vi "FFT.vi"() -> ()   [LabVIEW 2020]
uses:
  <vilib>/Platform/TimedLoop/XDataNode/timing_clust.ctl
  <vilib>/Platform/TimedLoop/XDataNode/nitl_modes.ctl
  <vilib>/Platform/TimedLoop/XDataNode/wakeup.ctl
  <vilib>/rvi/Analysis/measure/FFT/simModelSupport/niFPGA FFT Streaming Sim Properties.ctl
  <vilib>/rvi/Analysis/measure/FFT/simModelSupport/niFPGA FFT Sim Stream Group Properties.ctl
  <vilib>/rvi/Analysis/measure/FFT/simModelSupport/niFPGA FFT Sim Types.ctl
  <vilib>/rvi/Analysis/measure/FFT/simModelSupport/niFpgaFFTSimArithmeticProperties.ctl
  <vilib>/rvi/Analysis/measure/FFT/simModelSupport/niFpgaFFTSimDfxp.ctl
  <vilib>/fxp/LVFixedPointQuantizationPolicyTypeDef.ctl
  <vilib>/rvi/Analysis/measure/FFT/XNode/niFpgaFFTButterflyDelays.ctl
  <vilib>/rvi/DataTransferAndStorage/Container/Common/niFpgaContainerGetUniqueNameForEmu.vi
  <vilib>/rvi/DataTransferAndStorage/Container/Common/niFpgaContainerSetEmuInfo.vi
  <vilib>/rvi/eio/common/nirviEmuReportErrorAndStop.vi
  <vilib>/rvi/interface/RandomDataEmulation/niFpgaRandomDataHandleErrors.vi
  <vilib>/rvi/DataTransferAndStorage/Container/Common/niFpgaContainerExecOnDevCompGetState.vi
  <vilib>/rvi/Emulation/niFpgaEmulationIsFPGAContextNoSignature.vi
  <vilib>/rvi/Emulation/niFpgaSctlEmulationGetInTimedLoop.vi
  <vilib>/rvi/errors/niFpgaSetErrorForExecOnDevCompSimple.vi
  <vilib>/rvi/FIFO/Fifo_Resource/nirvififoEmulationSetSize.vi
  <vilib>/rvi/FIFO/Fifo_Resource/nirviFifoEmulationQueueMgr.vi
  <instcachedir>/0/nirviFifoEmulationQueueMgr_E5CAEC123FF24DC58D834DCA3CDAA9B5.lvgen/nirviFifoEmulationQueueMgr_E5CAEC123FF24DC58D834DCA3CDAA9B5_008.vi
  <vilib>/rvi/FIFO/Fifo_Resource/nirvififoEmulationDetermineInputValidOut.vi
  <vilib>/rvi/FIFO/Fifo_Resource/nirvififoEmulationCreateLock.vi
  <vilib>/rvi/Emulation/niFpgaProcessEmulError.vi
  <vilib>/rvi/FIFO/Fifo_Resource/nirvififoEmulationObtainLock.vi
  <vilib>/rvi/FIFO/Fifo_Resource/nirvififoEmulationReleaseLock.vi
  <vilib>/rvi/occurrence/nirviWaitOnOccurrenceBase.vi
  <vilib>/rvi/errors/nirviReportUnexpectedCaseInternalError.vi
  <vilib>/rvi/errors/nirviReportUnexpectedCaseInternalError (U32).vi
  <vilib>/Utility/error.llb/Clear Errors.vi
  <vilib>/rvi/Emulation/niFpgaEmulationReportErrorSimple.vi
  <vilib>/rvi/Emulation/niFpgaGetClockAttributes.vi
  <vilib>/rvi/Emulation/niFpgaCriticalErrorInLSC.vi
  <vilib>/rvi/Analysis/measure/FFT/simModelSupport/niFpgaFFTSimModelStreamingCore.vi
  <vilib>/rvi/LocalResourceManager/LocalResourceManager.xnode
  <vilib>/rvi/DataTransferAndStorage/Container/XNode/niFpgaContainer.xnode
  <vilib>/rvi/interface/RandomDataEmulation/nirviRandomDataFpgaReadWriteTemplate.vi
  <vilib>/rvi/FIFO/Fifo_Resource/niFpgaFifoEmulationRefIn.vi
  <vilib>/Platform/TimedLoop/XDataNode/XDataNode.xnode
  <vilib>/rvi/Analysis/measure/FFT/XNode/niFpgaFFT.xnode
  <vilib>/rvi/FXPMathLib/FxpInterpret/XNode/nifxpmath_Interpret.xnode
  <vilib>/Platform/TimedLoop/XDataNode/XDNodeRunTimeDep.lvlib
panel:
  out "overflow":bool
  out "loop numbers for FFT":i32
  out "loop number for data collection":i32
  out "appended array":fxp<+/-,24,7>[](array[numeric])
  out "FFT time (uSec)":u32
  out "data collection time (uSec)":u32
  in  "auto stop":bool
  in  "FFT loop iterations":i32
  out "Element":fxp<+/-,24,7>
  in  "Loop number":i32
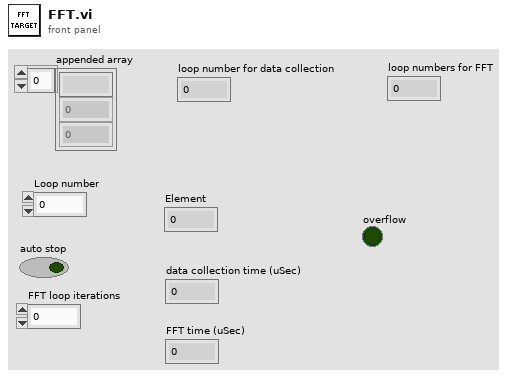
[diagram p1: front panel]
types:
  T1 = typedef "XDNodeRunTimeDep.lvlib/timing_clust.ctl" = cluster{"Expected End [f-1]":u64, "Actual End [f-1]":u64, "Finished Late? [f-1]":bool, "Expected End [i-1]":u64, "Actual End [i-1]":u64, "Finished Late? [i-1]":bool, "Expected Start [i]":u64, "Actual Start [i]":u64, "Expected Start [f]":u64, "Actual Start [f]":u64, "Source Name":string, "Structure Name":string, "Period":i64, "Deadline":i64, "Offset":i64, "Start":i64, "Priority":i32, "Timeout":i32, "Mode":T2, "Wakeup Reason":T3, "Error":errorcluster, "Source Type":string, "Secondary Source Type":string, "Global End Time":u64, "Global Start Time":u64, "Frame Duration":u64, "Iteration Duration":u64, "Assigned CPU":i32, "I/O Scan Engine Mode":u32}
  T2 = typedef "XDNodeRunTimeDep.lvlib/nitl_modes.ctl" = enum32{"No Change", "Process missed periods, maintain original phase", "Discard missed periods, maintain original phase", "Process missed periods, ignore original phase", "Discard missed periods, ignore original phase"}
  T3 = typedef "XDNodeRunTimeDep.lvlib/wakeup.ctl" = enum32{"Normal", "Aborted", "Asynchronous wakeup", "Timing source error", "Timed loop error", "Timeout"}
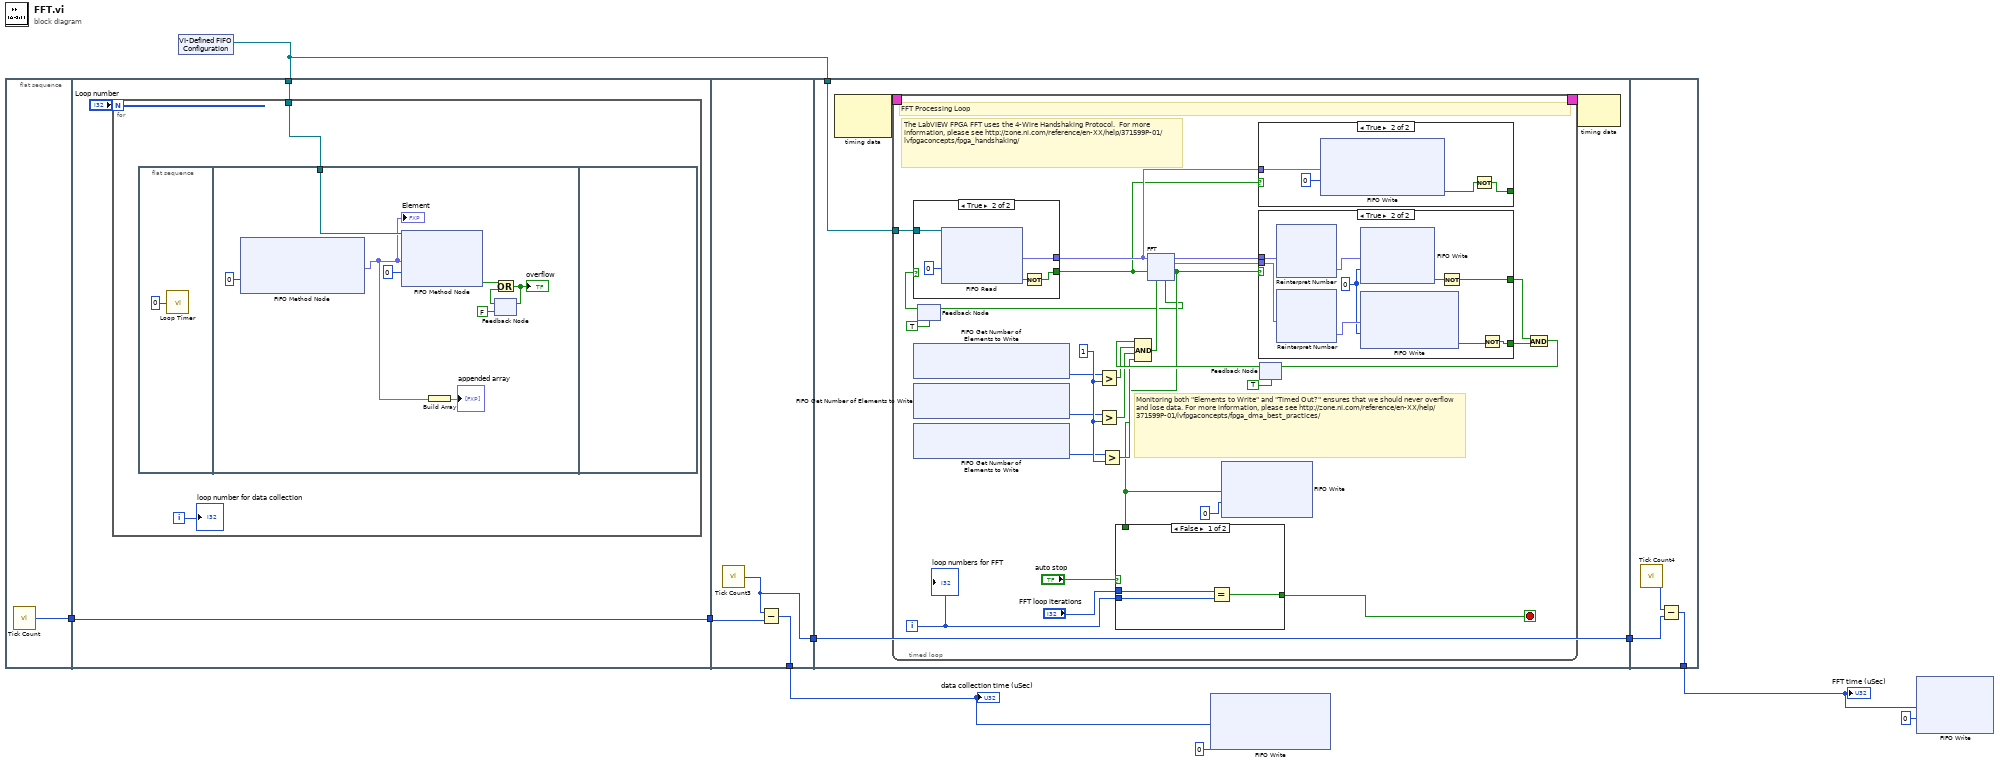
[diagram p0: block diagram]
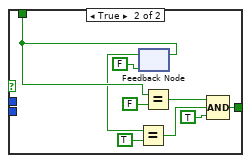
[diagram p2: hidden frame]
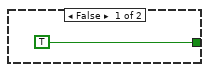
[diagram p3: hidden frame]
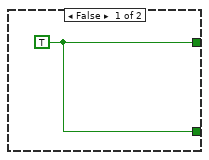
[diagram p4: hidden frame]
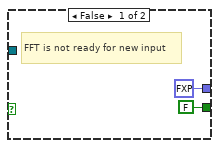
[diagram p5: hidden frame]
diagram:
  n1 = flat-sequence {
    tunnel: [w10] -> w9
    tunnel: w5 -> [w13]
    tunnel: w9 -> [w11]
    tunnel: [w11] -> w8
    tunnel: w8 -> [w28]
    tunnel: [w27] -> w4
    tunnel: [w26] -> w7
    tunnel: w5 -> [w30]
    tunnel: w7 -> [w29]
    tunnel: [w29] -> w6
    tunnel: w6 -> [w125]
    tunnel: [w124] -> w1
    frame #0 {
      n2 = call "Tick Count"() -> ("Tick Count(uSec)"=w10:u32)
    }
    frame #1 {
      n3 = for {
        N: "Loop number" -> [_]
        tunnel: w13 -> [w15]
        i -> [w14]
        n4 = flat-sequence {
          tunnel: w15 -> [w24]
          frame #0 {
            n5 = call "Loop Timer"("Count(mSec)"=u32 0) -> ()  [unwired: 1 out]
          }
          frame #1 {
            n6 = xnode ("FIFO Method Node")("Timeout"=0) -> ("Element"=w22:fxp<+/-,24,7>)  [unwired: 1 in, 2 out]
            "Element" <- w22
            n7 = xnode ("FIFO Method Node")("Element"=w22, "Timeout"=0, "FIFO In"=w24) -> ("Timed Out?"=w19:bool)  [unwired: 1 in, 2 out]
            n8 = Build Array(w22) -> (→"appended array":fxp<+/-,24,7>[])
            n9 = feedback #1(FALSE) -> (w18:bool)
            n10 = Or(x=w19, y=w18) -> (x .or. y?=w20:bool)
            "overflow" <- w20
            n11 = feedback-in #1(w20) -> ()
          }
          frame #2 {
          }
        }
        "loop number for data collection" <- w14
      }
    }
    frame #2 {
      n12 = call "Tick Count3"() -> ("Tick Count(uSec)"=w26:u32)
      n13 = Subtract(x=w26, y=w28) -> (x-y=w27:u32)
    }
    frame #3 {
      n14 = node-c288() -> (w32:T1)  [unwired: 2 in]
      n15 = timed-loop {
        timing: w32 -> [_]
        timing-out: [_] -> w31
        tunnel: w30 -> [w57]
        i -> [w34]
        stop <- w43 stop-if-true
        w52 = u32 1 ("y")
        # "Monitoring both \"Elements to Write\" and \"Timed Out?\" ensures that we should never overflow and lose data. For more information, please see http://zone.ni.com/reference/en-XX/help/371599P-01/lvfpgaconcepts/fpga_dma_best_practices/"
        # "The LabVIEW FPGA FFT uses the 4-Wire Handshaking Protocol.  For more information, please see http://zone.ni.com/reference/en-XX/help/371599P-01/lvfpgaconcepts/fpga_handshaking/"
        # "FFT Processing Loop"
        n16 = xnode ("FIFO Get Number of Elements to Write")() -> ("Number of Elements to Write"=w37:u32)  [unwired: 1 in, 1 out]
        n17 = xnode ("FIFO Get Number of Elements to Write")() -> ("Number of Elements to Write"=w36:u32)  [unwired: 1 in, 1 out]
        n18 = xnode ("FIFO Get Number of Elements to Write")() -> ("Number of Elements to Write"=w35:u32)  [unwired: 1 in, 1 out]
        n19 = feedback #2(TRUE ("ready for input")) -> (w59:bool)
        n20 = case shown="True" w59 {
          tunnel: [FALSE w118] -> w45
          tunnel: [fxp<+/-,16,5> 0.0 ("Element") w119] -> w58
          tunnel: w57 -> [_ w115]
          frame False {
            # "FFT is not ready for new input"
          }
          frame True {
            n21 = xnode ("FIFO Read")("Timeout"=0, "FIFO In"=w115) -> ("Element"=w119:fxp<+/-,24,7>, "Timed Out?"=w117:bool)  [unwired: 1 out]
            n22 = Not(x=w117) -> (.not. x?=w118:bool)
          }
        }
        n23 = Greater?(x=w37, y=w52) -> (0:w50:bool)
        n24 = Greater?(x=w36, y=w52) -> (0:w49:bool)
        n25 = Greater?(x=w35, y=w52) -> (0:w48:bool)
        n26 = case shown="True" w45 {
          tunnel: w58 -> [_ w73]
          tunnel: [TRUE ("Timed Out?") w74] -> _
          frame False {
          }
          frame True {
            n27 = xnode ("FIFO Write")("Element"=w73, "Timeout"=0) -> ("Timed Out?"=w75:bool)  [unwired: 1 in, 1 out]
            n28 = Not(x=w75) -> (.not. x?=w74:bool)
          }
        }
        n29 = feedback #3(TRUE) -> (w51:bool)
        n30 = Compound Arithmetic op=AND(w51, w50, w49, w48) -> (w44:bool)
        n31 = xnode "FFT"("real data in"=w58, "input valid"=w45, "ready for output"=w44) -> ("ready for input"=w33:bool, "real data out"=w56:fxp<+/-,32,15>, "imaginary data out"=w42:fxp<+/-,32,15>, "output valid"=w39:bool)  [unwired: 2 in, 1 out]
        n32 = feedback-in #2(w33) -> ()
        n33 = case shown="False" "auto stop" {
          tunnel: w39 -> [_ w70]
          tunnel: [w60 w63] -> w43
          tunnel: w34 -> [w62 _]
          tunnel: "FFT loop iterations" -> [w61 _]
          frame False {
            n34 = Equal?(x=w61, y=w62) -> (x = y?=w60:bool)
          }
          frame True {
            n35 = feedback #4(FALSE) -> (w67:bool)
            n36 = Equal?(x=w67, y=TRUE) -> (x = y?=w65:bool)
            n37 = feedback-in #4(w70) -> ()
            n38 = Equal?(x=w70, y=FALSE) -> (x = y?=w66:bool)
            n39 = Compound Arithmetic op=AND(w66, w65, TRUE ("value")) -> (w63:bool)
          }
        }
        n40 = xnode ("FIFO Write")("Element"=w39, "Timeout"=0) -> ()  [unwired: 1 in, 2 out]
        n41 = case shown="True" w39 {
          tunnel: w56 -> [_ w110]
          tunnel: w42 -> [_ w109]
          tunnel: [w103 w112] -> w55
          tunnel: [w103 w111] -> w54
          frame False {
            w103 = TRUE ("Timed Out?")
          }
          frame True {
            w106 = 0 ("Timeout")
            n42 = xnode "Reinterpret Number"("x"=w110) -> ("y"=w108:fxp<+/-,32,21>)
            n43 = xnode "Reinterpret Number"("x"=w109) -> ("y"=w107:fxp<+/-,32,21>)
            n44 = xnode ("FIFO Write")("Element"=w108, "Timeout"=w106) -> ("Timed Out?"=w105:bool)  [unwired: 1 in, 1 out]
            n45 = xnode ("FIFO Write")("Element"=w107, "Timeout"=w106) -> ("Timed Out?"=w104:bool)  [unwired: 1 in, 1 out]
            n46 = Not(x=w105) -> (.not. x?=w112:bool)
            n47 = Not(x=w104) -> (.not. x?=w111:bool)
          }
        }
        n48 = Compound Arithmetic op=AND(w55, w54) -> (w46:bool)
        n49 = feedback-in #3(w46) -> ()
        "loop numbers for FFT" <- w34
      }
      n50 = node-c288(w31) -> ()  [unwired: 1 out]
    }
    frame #4 {
      n51 = call "Tick Count4"() -> ("Tick Count(uSec)"=w126:u32)
      n52 = Subtract(x=w126, y=w125) -> (x-y=w124:u32)
    }
  }
  n53 = xnode "VI-Defined FIFO Configuration"() -> ("FIFO Out"=w5:refnum<k21>)
  n54 = xnode ("FIFO Write")("Element"=w4, "Timeout"=0) -> ()  [unwired: 1 in, 2 out]
  n55 = xnode ("FIFO Write")("Element"=w1, "Timeout"=0) -> ()  [unwired: 1 in, 2 out]
  "data collection time (uSec)" <- w4
  "FFT time (uSec)" <- w1
